vi "Serialize - Text.vi"(8 "error in":errorcluster, 11 "Data in":refnum<class "Data.lvclass">) -> (0 "error out":errorcluster, 2 "Serialized Text":string, 3 "Data out":refnum<class "Data.lvclass">)   [LabVIEW 2014, in "Base Data Class.lvlib" / "Data.lvclass"]
uses:
  Data.lvclass
  Data.lvclass/Data.ctl
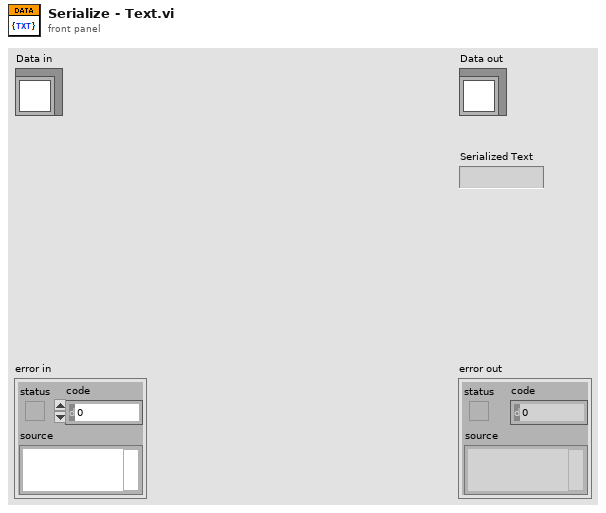
[diagram p1: front panel]
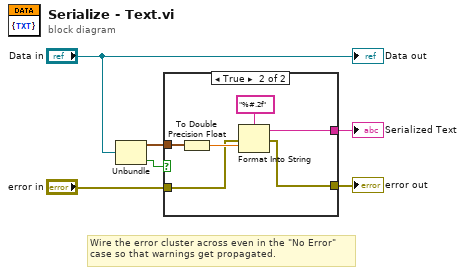
[diagram p0: block diagram]
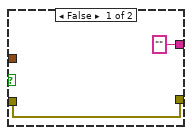
[diagram p2: hidden frame]
diagram:
  # "Wire the error cluster across even in the \"No Error\"\ncase so that warnings get propagated."
  n1 = Unbundle("Data in") -> (w4:timestamp, w1:bool)  [unwired: 1 out]
  n2 = case shown="True" w1 {
    tunnel: ["" w14] -> w5
    tunnel: w4 -> [_ w13]
    tunnel: "error in" -> [w7 w10]
    tunnel: [w7 w9] -> w2
    frame False {
    }
    frame True {
      n3 = To Double Precision Float(number=w13) -> (double precision float=w12:dbl)
      n4 = Format Into String(format string="%#.2f", error in=w10, w12) -> (resulting string=w14:string, error out=w9:errorcluster)  [unwired: 1 in]
    }
  }
  "error out" <- w2
  "Serialized Text" <- w5
  "Data out" <- "Data in"
